vi "HT Voting (SubVI).vi"(7 "Max Vote":i16=5, 9 "Larvae Index":i32, 10 "Negative Vote":bool, 11 "Positive Vote":bool) -> (0 "Vote Array":i16[](array[numeric]), 3 "Vote Valid?":bool)   [LabVIEW 2015]
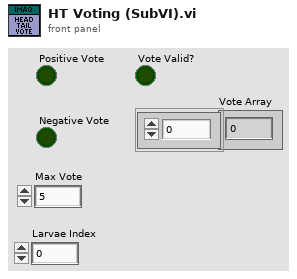
[diagram p1: front panel]
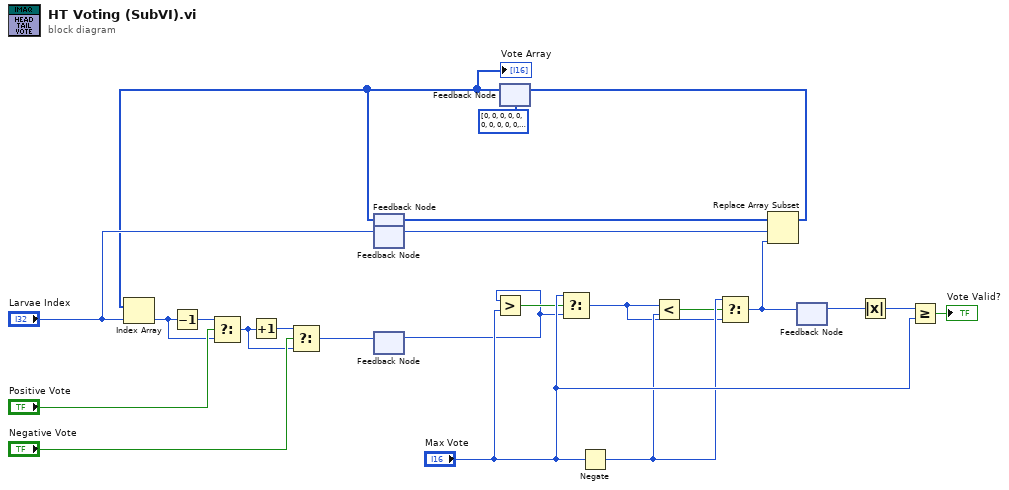
[diagram p0: block diagram]
diagram:
  n1 = feedback #1() -> (w2:i16[])  [unwired: 1 in]
  n2 = feedback-in #2("Larvae Index") -> ()
  n3 = feedback #2() -> (w3:i32)  [unwired: 1 in]
  n4 = feedback #3() -> (w4:i16)  [unwired: 1 in]
  n5 = Greater?(x=w4, y="Max Vote") -> (0:w13:bool)
  n6 = feedback #4(i16[] [0, 0, 0, 0, 0, 0, 0, 0, 0, 0, 0, 0, 0, 0, 0, 0]) -> (w1:i16[])
  "Vote Array" <- w1
  n7 = Index Array(array=w1, index="Larvae Index") -> (element=w8:i16)
  n8 = Decrement(x=w8) -> (x-1=w10:i16)
  n9 = Select(t=w10, s="Positive Vote", f=w8) -> (s? t:f=w12:i16)
  n10 = Increment(x=w12) -> (x+1=w11:i16)
  n11 = Select(t=w11, s="Negative Vote", f=w12) -> (s? t:f=w14:i16)
  n12 = feedback-in #1(w1) -> ()
  n13 = feedback-in #3(w14) -> ()
  n14 = Select(t="Max Vote", s=w13, f=w4) -> (s? t:f=w16:i16)
  n15 = Negate(x="Max Vote") -> (-x=w17:i16)
  n16 = Less?(x=w16, y=w17) -> (x < y?=w15:bool)
  n17 = Select(t=w17, s=w15, f=w16) -> (s? t:f=w6:i16)
  n18 = Replace Array Subset(array=w2, new element=w6, index=w3) -> (w5:i16[])
  n19 = feedback-in #4(w5) -> ()
  n20 = feedback #5() -> (w21:i16)  [unwired: 1 in]
  n21 = feedback-in #5(w6) -> ()
  n22 = Absolute Value(x=w21) -> (abs(x)=w18:i16)
  n23 = Greater Or Equal?(x=w18, y="Max Vote") -> (x >= y?=→"Vote Valid?":bool)
